vi "MH_DeInitDone.vi"(8 "error in (no error)":errorcluster, 11 "MultiharpComm in":refnum<class "MultiharpComm.lvclass">) -> (0 "error out":errorcluster, 3 "MultiharpComm out":refnum<class "MultiharpComm.lvclass">)   [LabVIEW 2023, in "SinglePhoton Library.lvlib" / "MultiharpComm.lvlib" / "MultiharpComm.lvclass"]
uses:
  MultiharpComm.lvclass
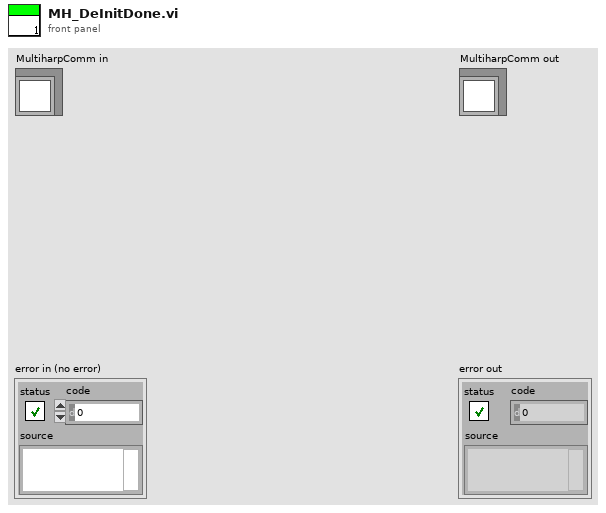
[diagram p1: front panel]
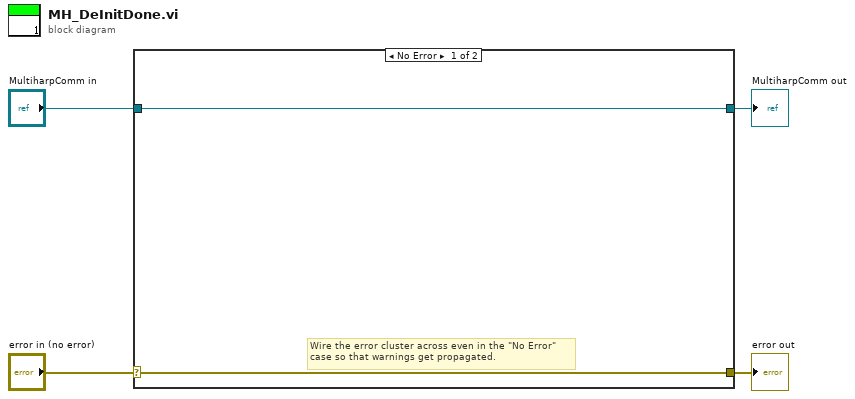
[diagram p0: block diagram]
diagram:
  n1 = case shown="No Error" "error in (no error)" {
    selector: "error in (no error)" -> [w5 w8]
    tunnel: [w5 w8] -> w3
    tunnel: [w6 w7] -> w1
    tunnel: "MultiharpComm in" -> [w6 w7]
    frame No Error {
      # "Wire the error cluster across even in the \"No Error\"\ncase so that warnings get propagated."
    }
    frame Error {
    }
  }
  "error out" <- w3
  "MultiharpComm out" <- w1
